vi "getcurrent.vi"(5 "forcemode":i32, 6 "maxcurrentin":dbl, 7 "setpoint":dbl, 9 "minforcey":dbl, 10 "maxforcey":dbl, 11 "currentin":dbl) -> ()   [LabVIEW 2017, in "HapticSTM.lvlib"]
doc: "extern \"C\" __declspec(dllexport) void getcurrent(double currentin, double maxforcey, double minforcey, double setpoint, double maxcurrentin, int forcemode);"
uses:
  <userlib>/HapticSTM/Feedbackless - Testdata/Yscalingtest Folder/HapticSTM.lvlib
  <userlib>/HapticSTM/HapticSTM.dll
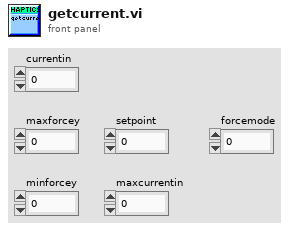
[diagram p1: front panel]
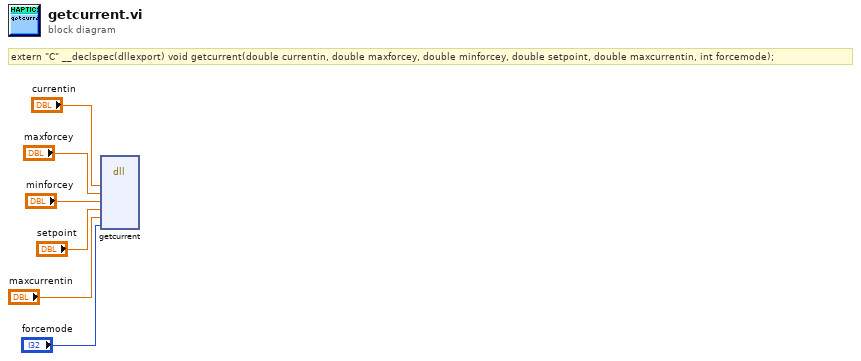
[diagram p0: block diagram]
diagram:
  # "extern \"C\" __declspec(dllexport) void getcurrent(double currentin, double maxforcey, double minforcey, double setpoint, double maxcurrentin, int forcemode);"
  n1 = dll-call lib="C:/Program Files/National Instruments/LabVIEW 2019/user.lib/HapticSTM/HapticSTM.*" fn="getcurrent"("currentin"="currentin", "maxforcey"="maxforcey", "minforcey"="minforcey", "setpoint"="setpoint", "maxcurrentin"="maxcurrentin", "forcemode"="forcemode") -> ()  [unwired: 10 in, 2 out]
